vi "Read Starting Temperature.vi"(11 "thermal test in":refnum<class "Thermal Test.lvclass">) -> (1 "starting temperature":dbl[unit]=273.15)   [LabVIEW 2023, in "Thermal Test.lvclass"]
uses:
  Thermal Test.lvclass
  Thermal Test.lvclass/Thermal Test.ctl
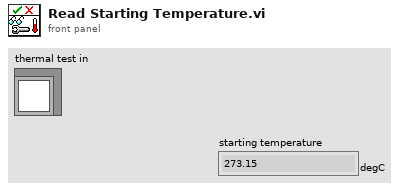
[diagram p1: front panel]
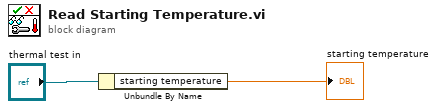
[diagram p0: block diagram]
diagram:
  n1 = Unbundle By Name("thermal test in") -> ("starting temperature"=→"starting temperature":dbl[unit])
